vi "IsFolderDotGit.vi"(8 "error in":errorcluster, 11 "path":path) -> (0 "error out":errorcluster, 3 "Is .git folder":bool)   [LabVIEW 2018, in "feGEM DataPacker.lvlib"]
uses:
  feGEM DataPacker.lvlib
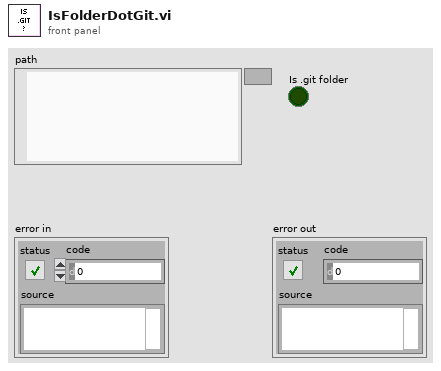
[diagram p1: front panel]
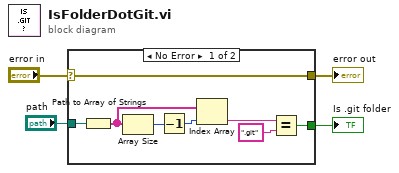
[diagram p0: block diagram]
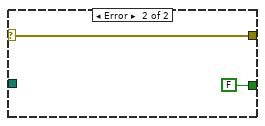
[diagram p2: hidden frame]
diagram:
  n1 = case shown="No Error" "error in" {
    selector: "error in" -> [w5 w13]
    tunnel: [w7 FALSE] -> w4
    tunnel: "path" -> [w6 _]
    tunnel: [w5 w13] -> w1
    frame No Error {
      n2 = Path to Array of Strings(0:w6) -> (2:w12:string[])  [unwired: 1 out]
      n3 = Array Size(array=w12) -> (size(s)=w11:i32)
      n4 = Decrement(x=w11) -> (x-1=w10:i32)
      n5 = Index Array(array=w12, index=w10) -> (element=w9:string)
      n6 = Equal?(x=w9, y=".git") -> (x = y?=w7:bool)
    }
    frame Error {
    }
  }
  "Is .git folder" <- w4
  "error out" <- w1
